vi "vector_v3.vi"() -> ()   [LabVIEW 2009]
panel:
  in  "stop":bool
  out "Elementul selectat":dbl=235.0
  in  "Index":u8(slide)=5 scale=9.0..0.0
  in  "Vector cu elemente numerice":dbl[](array[numeric])=[123.0, 646.0, 567.0, 16.0, 23454.0, 235.0, 45445.0, 45.0, 45.0, 90.0]
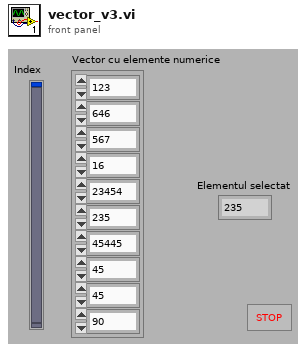
[diagram p1: front panel]
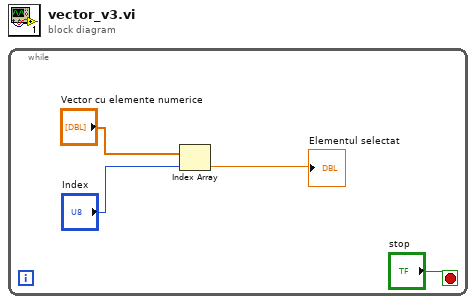
[diagram p0: block diagram]
diagram:
  n1 = while {
    stop <- "stop" stop-if-true
    n2 = Index Array(array="Vector cu elemente numerice", index="Index") -> (element=→"Elementul selectat":dbl)
  }
